vi "Save Inputs.vi"(10 "error in":errorcluster, 11 "DesignRequest":T2={"Project Folder"=path "D:/inetpub/wwwroot/Designs/EtFlocSedFi/5174/342584978976", "Method Name"="EtFlocSedFi", "Inputs"=[{"Label.Text"="UI.Name", "Control Type"=4, "Numeric"=0.0, "Array"=[], "status"=FALSE, "Str Array"=[], "String"="Monroe Weber-Shirk", "unit"=""}, {"Label.Text"="UI.Email", "Control Type"=4, "Numeric"=0.0, "Array"=[], "status"=FALSE, "Str Array"=[], "String"="mw24@cornell.edu", "unit"=""}, {"Label.Text"="UI.Organization", "Control Type"=4, "Numeric"=0.0, "Array"=[], "status"=FALSE, "Str Array"=[], "String"="Cornell University", "unit"=""}, {"Label.Text"="UI.Country", "Control Type"=4, "Numeric"=0.0, "Array"=[], "status"=FALSE, "Str Array"=[], "String"="US", "unit"=""}, {"Label.Text"="UI.ProjectTitle", "Control Type"=4, "Numeric"=0.0, "Array"=[], "status"=FALSE, "Str Array"=[], "String"="12 L/s plant", "unit"=""}, {"Label.Text"="UI.ProjectCity", "Control Type"=4, "Numeric"=0.0, "Array"=[], "status"=FALSE, "Str Array"=[], "String"="ITHACA", "unit"=""}, {"Label.Text"="UI.ProjectState", "Control Type"=4, "Numeric"=0.0, "Array"=[], "status"=FALSE, "Str Array"=[], "String"="New York", "unit"=""}, {"Label.Text"="UI.ProjectNotes", "Control Type"=4, "Numeric"=0.0, "Array"=[], "status"=FALSE, "Str Array"=[], "String"="", "unit"=""}, {"Label.Text"="Q.Plant", "Control Type"=18, "Numeric"=18.0, "Array"=[], "status"=FALSE, "Str Array"=[], "String"="", "unit"="L/s"}], "Version"=5174}) -> (2 "error out":errorcluster)   [LabVIEW 2012]
uses:
  Design Request.ctl
  Variable cluster.ctl
  Design Server.lvlib
panel:
  out "sorted array":T1
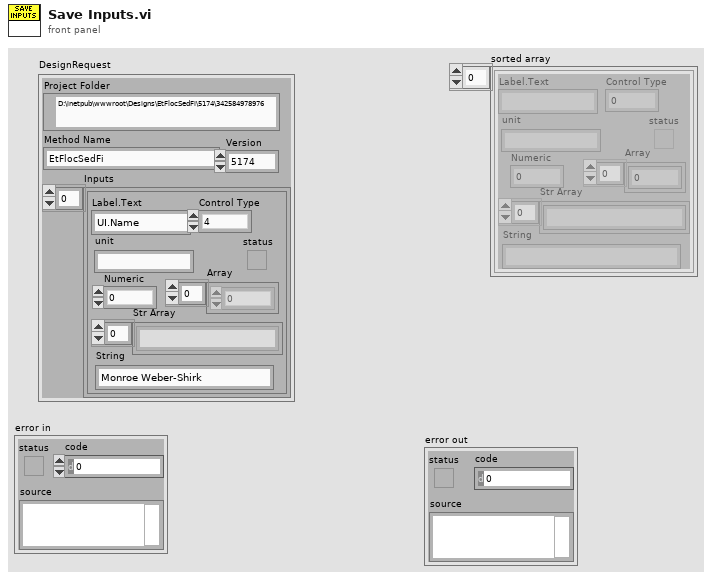
[diagram p1: front panel]
types:
  T1 = typedef "Design Server.lvlib/Variable cluster.ctl" = cluster{"Label.Text":string, "Control Type":u32, "Numeric":dbl, "Array":dbl[], "status":bool, "Str Array":string[], "String":string, "unit":string}[]
  T2 = typedef "Design Server.lvlib/Design Request.ctl" = cluster{"Project Folder":path, "Method Name":string, "Inputs":T1, "Version":i32}
  T3 = cluster{"Label.Text":string, "Control Type":u32, "Numeric":dbl, "Array":dbl[], "status":bool, "Str Array":string[], "String":string, "unit":string}[]
  T4 = enum16{"open", "replace", "create", "open or create", "replace or create", "replace or create with confirmation"}
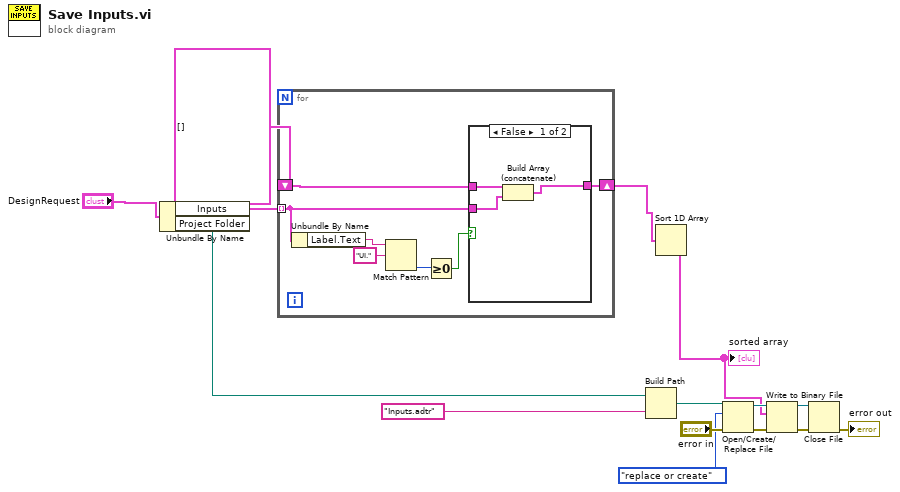
[diagram p0: block diagram]
diagram:
  n1 = Unbundle By Name("DesignRequest") -> ("Inputs"=w3:T1, "Project Folder"=w6:path)
  n2 = for {
    tunnel: w3 -> [w16] mode=indexing
    shift-right: [w18] -> w1
    shift-left: T3 [] -> [w17]
    n3 = Unbundle By Name(w16) -> ("Label.Text"=w22:string)
    n4 = Match Pattern(string=w22, regular expression="UI.") -> (offset past match=w20:i32)  [unwired: 1 in, 3 out]
    n5 = Greater Or Equal To 0?(x=w20) -> (x >= 0?=w19:bool)
    n6 = case shown="False" w19 {
      tunnel: [w24 w26] -> w18
      tunnel: w17 -> [w23 w26]
      tunnel: w16 -> [w25 _]
      frame False {
        n7 = Build Array (concatenate)(w23, w25) -> (w24:T3)
      }
      frame True {
      }
    }
  }
  n8 = Build Path(base path=w6, name or relative path="Inputs.adtr") -> (appended path=w11:path)
  n9 = Sort 1D Array(array=w1) -> (sorted array=w4:T3)
  "sorted array" <- w4
  n10 = Open/Create/Replace File(file path (use dialog)=w11, error in="error in", operation (0:open)=T4."replace or create") -> (refnum out=w14:refnum<file>, error out=w15:errorcluster)  [unwired: 3 in, 1 out]
  n11 = Write to Binary File(file (use dialog)=w14, data=w4, error in=w15) -> (refnum out=w13:refnum<file>, error out=w12:errorcluster)  [unwired: 3 in, 1 out]
  n12 = Close File(refnum=w13, error in=w12) -> (error out=→"error out":errorcluster)  [unwired: 1 out]
